vi "探头校准标准值设置.vi"(7 "校准参数":u16(ring) caption="校准参数：" items=["pH", "DO", "浊度", "电导率", "叶绿素a", "藻密度", "ORP", "DO2"], 9 "标液三":sgl, 10 "标液二":sgl, 11 "标液一":sgl) -> ()   [LabVIEW 2016, in "斯坦道多参数.lvlib"]
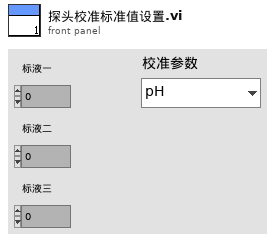
[diagram p1: front panel]
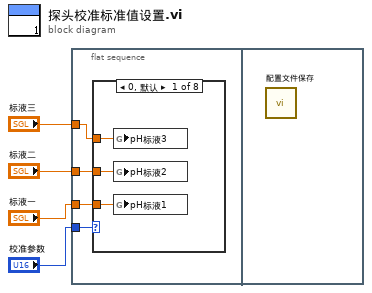
[diagram p0: block diagram]
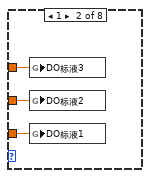
[diagram p2: hidden frame]
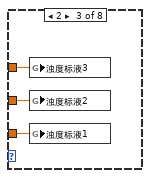
[diagram p3: hidden frame]
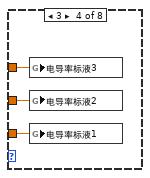
[diagram p4: hidden frame]
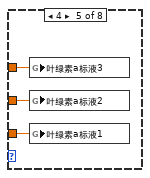
[diagram p5: hidden frame]
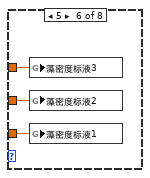
[diagram p6: hidden frame]
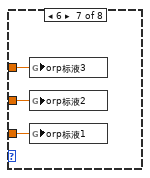
[diagram p7: hidden frame]
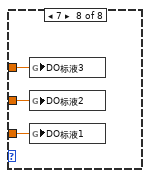
[diagram p8: hidden frame]
diagram:
  n1 = flat-sequence {
    tunnel: "校准参数" -> [w8]
    tunnel: "标液一" -> [w7]
    tunnel: "标液二" -> [w6]
    tunnel: "标液三" -> [w5]
    frame #0 {
      n2 = case shown="0, 默认" w8 {
        tunnel: w7 -> [w11 w14 w17 w20 w23 w26 w29 w32]
        tunnel: w6 -> [w10 w13 w16 w19 w22 w25 w28 w31]
        tunnel: w5 -> [w9 w12 w15 w18 w21 w24 w27 w30]
        frame 0, Default {
          n3 = global write "断电保存变量.vi" "pH标液3"(w9) -> ()
          n4 = global write "断电保存变量.vi" "pH标液2"(w10) -> ()
          n5 = global write "断电保存变量.vi" "pH标液1"(w11) -> ()
        }
        frame 1 {
          n6 = global write "断电保存变量.vi" "DO标液3"(w12) -> ()
          n7 = global write "断电保存变量.vi" "DO标液2"(w13) -> ()
          n8 = global write "断电保存变量.vi" "DO标液1"(w14) -> ()
        }
        frame 2 {
          n9 = global write "断电保存变量.vi" "浊度标液3"(w15) -> ()
          n10 = global write "断电保存变量.vi" "浊度标液2"(w16) -> ()
          n11 = global write "断电保存变量.vi" "浊度标液1"(w17) -> ()
        }
        frame 3 {
          n12 = global write "断电保存变量.vi" "电导率标液3"(w18) -> ()
          n13 = global write "断电保存变量.vi" "电导率标液2"(w19) -> ()
          n14 = global write "断电保存变量.vi" "电导率标液1"(w20) -> ()
        }
        frame 4 {
          n15 = global write "断电保存变量.vi" "叶绿素a标液3"(w21) -> ()
          n16 = global write "断电保存变量.vi" "叶绿素a标液2"(w22) -> ()
          n17 = global write "断电保存变量.vi" "叶绿素a标液1"(w23) -> ()
        }
        frame 5 {
          n18 = global write "断电保存变量.vi" "藻密度标液3"(w24) -> ()
          n19 = global write "断电保存变量.vi" "藻密度标液2"(w25) -> ()
          n20 = global write "断电保存变量.vi" "藻密度标液1"(w26) -> ()
        }
        frame 6 {
          n21 = global write "断电保存变量.vi" "orp标液3"(w27) -> ()
          n22 = global write "断电保存变量.vi" "orp标液2"(w28) -> ()
          n23 = global write "断电保存变量.vi" "orp标液1"(w29) -> ()
        }
        frame 7 {
          n24 = global write "断电保存变量.vi" "DO标液3"(w30) -> ()
          n25 = global write "断电保存变量.vi" "DO标液2"(w31) -> ()
          n26 = global write "断电保存变量.vi" "DO标液1"(w32) -> ()
        }
      }
    }
    frame #1 {
      n27 = call "配置文件保存.vi"() -> ()  [unwired: 12 in]
    }
  }
